vi "sinyal_gen_test.vi"(6 "Amplitude(V)":fxp<+,64,32>=1.0, 7 "Frequency(max:12.5MHz)":fxp<+,12,10>=1.0, 8 "OFFSET":bool, 9 "OUTPUT":bool) -> ()   [LabVIEW 2016]
uses:
  <vilib>/Instr/_visa.llb/VISA Configure Serial Port (Instr).vi
panel:
  in  "Signal Gen Port":refnum<visa-resource-name>="COM4"
  in  "Frequency Type":string(combo)="kHz"
  in  "Offset Set(V)":dbl=0.1
  in  "Wave Type":T1(radio)
  in  "stop":bool
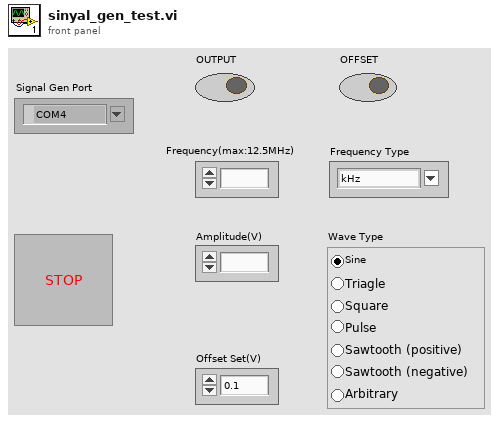
[diagram p1: front panel]
types:
  T1 = enum32{"Sine", "Triagle", "Square", "Pulse", "Sawtooth (positive)", "Sawtooth (negative)", "Arbitrary"}
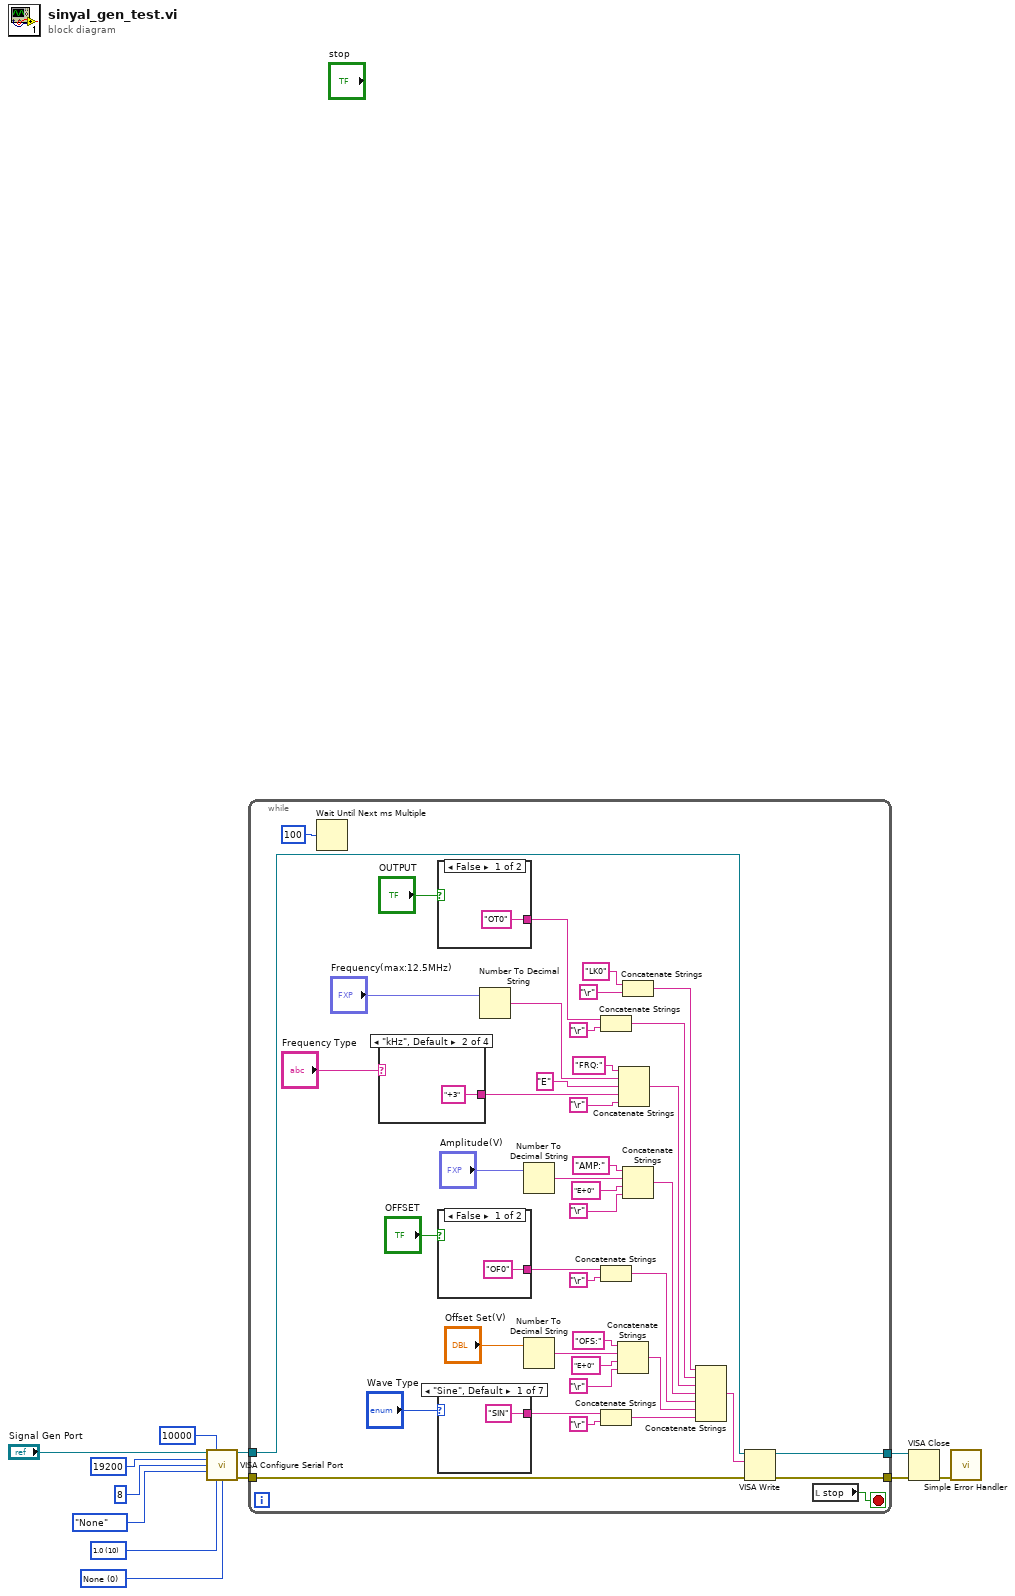
[diagram p0: block diagram]
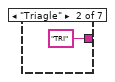
[diagram p2: hidden frame]
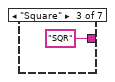
[diagram p3: hidden frame]
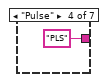
[diagram p4: hidden frame]
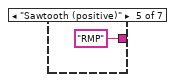
[diagram p5: hidden frame]
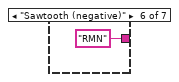
[diagram p6: hidden frame]
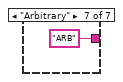
[diagram p7: hidden frame]
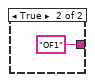
[diagram p8: hidden frame]
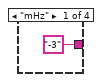
[diagram p9: hidden frame]
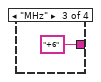
[diagram p10: hidden frame]
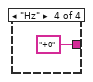
[diagram p11: hidden frame]
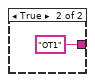
[diagram p12: hidden frame]
diagram:
  w12 = u16 0 items=["None", "XON/XOFF", "RTS/CTS", "XON/XOFF & RTS/CTS", "DTR/DSR", "XON/XOFF & DTR/DSR"] ("flow control (0:none)")
  w11 = u16 10 items=["1.0"=10, "1.5"=15, "2.0"=20] ("stop bits (10: 1 bit)")
  n1 = call-poly "VISA Configure Serial Port"("VISA resource name"="Signal Gen Port", "timeout (10sec)"=u32 10000, "baud rate (9600)"=u32 19200, "data bits (8)"=u16 8, "parity (0:none)"=enum16{"None", "Odd", "Even", "Mark", "Space"}."None", "stop bits (10: 1 bit)"=w11, "flow control (0:none)"=w12) -> ("VISA resource name out"=w6:refnum<visa-resource-name>, "error out"=w5:errorcluster)  [unwired: 7 in]
  n2 = while {
    tunnel: [w54] -> w2
    tunnel: [w53] -> w3
    tunnel: w6 -> [w15]
    tunnel: w5 -> [w14]
    stop <- w51 stop-if-true
    n3 = Wait Until Next ms Multiple(millisecond multiple=u32 100) -> ()  [unwired: 1 out]
    n4 = case shown="\"kHz\", Default" "Frequency Type" {
      tunnel: ["-3" "+3" "+6" "+0"] -> w47
      frame "mHz" {
      }
      frame "kHz", Default {
      }
      frame "MHz" {
      }
      frame "Hz" {
      }
    }
    n5 = case shown="False" "OUTPUT" {
      tunnel: ["OT0" "OT1"] -> w18
      frame False {
      }
      frame True {
      }
    }
    n6 = case shown="False" "OFFSET" {
      tunnel: ["OF0" "OF1"] -> w36
      frame False {
      }
      frame True {
      }
    }
    n7 = case shown="\"Sine\", Default" "Wave Type" {
      tunnel: ["SIN" "TRI" "SQR" "PLS" "RMP" "RMN" "ARB"] -> w44
      frame "Sine", Default {
      }
      frame "Triagle" {
      }
      frame "Square" {
      }
      frame "Pulse" {
      }
      frame "Sawtooth (positive)" {
      }
      frame "Sawtooth (negative)" {
      }
      frame "Arbitrary" {
      }
    }
    n8 = Number To Decimal String(number="Frequency(max:12.5MHz)") -> (decimal integer string=w23:string)  [unwired: 1 in]
    n9 = Number To Decimal String(number="Amplitude(V)") -> (decimal integer string=w30:string)  [unwired: 1 in]
    n10 = Number To Decimal String(number="Offset Set(V)") -> (decimal integer string=w41:string)  [unwired: 1 in]
    n11 = Concatenate Strings(w18, "\r") -> (w21:string)
    n12 = Concatenate Strings(w36, "\r") -> (w38:string)
    n13 = Concatenate Strings(w44, "\r") -> (w45:string)
    n14 = Concatenate Strings("OFS:", w41, "E+0", "\r") -> (w42:string)
    n15 = Concatenate Strings("FRQ:", w23, "E", w47, "\r") -> (w24:string)
    n16 = Concatenate Strings("LK0", "\r") -> (w20:string)
    n17 = Concatenate Strings("AMP:", w30, "E+0", "\r") -> (w31:string)
    n18 = Concatenate Strings(w20, w21, w24, w31, w38, w42, w45) -> (w13:string)
    n19 = VISA Write(VISA resource name=w15, write buffer=w13, error in (no error)=w14) -> (VISA resource name out=w54:refnum<visa-resource-name>, error out=w53:errorcluster)  [unwired: 1 out]
    n20 = local read "stop"() -> (w51:bool)
  }
  n21 = VISA Close(VISA resource name=w2, error in (no error)=w3) -> (error out=w4:errorcluster)
  n22 = call <vilib>:"Simple Error Handler.vi"("error in (no error)"=w4) -> ()  [unwired: 4 in, 5 out]
